vi "CapacitanceNavigation v2.1.vi"() -> ()   [LabVIEW 2021]
uses:
  <userlib>/Nanonis Prog Interface V5/Nanonis Prog Interface.lvlib
panel:
  in  "Z Frequency (Hz)":sgl=261.0
  in  "Z- Delta cap threshold (pA)":dbl=0.1
  in  "Z Amplitude (V)":sgl=260.0
  out "Delta reached?":bool
  out "Cap reached?":bool
  in  "Cap threshold (pA)":dbl
  in  "Z+ Delta cap threshold (pA)":dbl
  in  "pause":bool
  in  "Delete First Entry":bool
  in  "Time between averages (ms)":u32
  out "Avg index":i32=49
  in  "Averages":i32=50
  in  "milliseconds to wait":u32=1000
  in  "stop":bool
  in  "?":bool
  in  "Max Steps":u16=500
  in  "Direction":enum16{"X +", "X -", "Y +", "Y -", "Z +", "Z -"}(ring)=enum."Z +"
  out "Delta":cluster{"index":i32, sgl}[](graph)=[{"index"=100, -1.3574829}, {"index"=200, -1.4841919}, {"index"=300, -1.576477}, {"index"=400, -1.5935059}, {"index"=500, -1.618042}, {"index"=600, -1.6258545}, {"index"=700, -1.5469971}, {"index"=800, -1.4503174}, {"index"=900, -1.5161133}, {"index"=1000, -1.3947754}, {"index"=1100, -1.4649048}, {"index"=1200, -1.3322754}, {"index"=1300, -1.392456}, {"index"=1400, -1.2904053}, {"index"=1500, -1.291626}, {"index"=1600, -1.2921143}, {"index"=1700, -1.2836304}, {"index"=1800, -1.3444824}, {"index"=1900, -1.2155762}, {"index"=2000, -1.2328491}, {"index"=2100, -1.2090454}, {"index"=2200, -1.2058716}, {"index"=2300, -1.2508545}, {"index"=2400, -1.2296753}, {"index"=2500, -1.1306152}, {"index"=2600, -1.2440186}, {"index"=2700, -1.1461792}, {"index"=2800, -1.2349854}, {"index"=2900, -1.125}, {"index"=3000, -1.1894531}, {"index"=3100, -1.1911011}, {"index"=3200, -1.1334229}, {"index"=3300, -1.2139282}, {"index"=3400, -1.0455322}, {"index"=3500, -1.1482544}, {"index"=3600, -1.1663208}, {"index"=3700, -1.1547852}, {"index"=3800, -1.1334229}, {"index"=3900, -1.1394043}, {"index"=4000, -1.1153564}, {"index"=4100, -1.1187744}, {"index"=4200, -1.1342163}, {"index"=4300, -1.1434326}, {"index"=4400, -1.0510864}, {"index"=4500, -1.0391235}, {"index"=4600, -1.0696411}, {"index"=4700, -1.050354}, {"index"=4800, -1.09552}, {"index"=4900, -1.0064087}, {"index"=5000, -1.0879517}, {"index"=5100, -1.0756836}, {"index"=5200, -1.064331}, {"index"=5300, -1.0778809}, {"index"=5400, -1.0646973}, {"index"=5500, -1.0031738}, {"index"=5600, -1.0564575}, {"index"=5700, -1.0297852}, {"index"=5800, -0.9793091}, {"index"=5900, -1.0583496}, {"index"=6000, -1.0194702}, {"index"=6100, -0.9897461}, {"index"=6200, -0.99768066}, {"index"=6300, -1.0195312}, {"index"=6400, -0.9753418}, {"index"=6500, -1.0460205}, {"index"=6600, -0.9507446}, {"index"=6700, -0.9986572}, {"index"=6800, -0.9227295}, {"index"=6900, -0.90026855}, {"index"=7000, -0.96069336}, {"index"=7100, -0.92089844}, {"index"=7200, -0.9293823}, {"index"=7300, -0.85827637}, {"index"=7400, -0.94433594}, {"index"=7500, -0.8942871}, {"index"=7600, -0.91204834}, {"index"=7700, -0.9284668}, {"index"=7800, -0.994812}, {"index"=7900, -0.89501953}, {"index"=8000, -0.880188}, {"index"=8100, -0.95428467}, {"index"=8200, -0.8895874}, {"index"=8300, -0.951355}, {"index"=8400, -0.94384766}, {"index"=8500, -0.9460449}, {"index"=8600, -0.9188843}, {"index"=8700, -0.94177246}, {"index"=8800, -0.9863281}, {"index"=8900, -0.85375977}, {"index"=9000, -0.9229126}, {"index"=9100, -0.90771484}, {"index"=9200, -0.9472046}, {"index"=9300, -0.8875122}, {"index"=9400, -0.84661865}, {"index"=9500, -0.91223145}, {"index"=9600, -0.8786621}, {"index"=9700, -0.80389404}, {"index"=9800, -0.36602783}, {"index"=9900, 0.0076904297}, {"index"=10000, 0.010681152}, {"index"=10100, 0.0065307617}, {"index"=10200, -0.048583984}, {"index"=10300, 0.057373047}, {"index"=10400, 6.1035156e-05}, {"index"=10500, -0.085876465}]
  in  "Number of Steps":u16=100
  out "Capacitance":cluster{"index":i32, sgl}[](graph)=[{"index"=0, 783.6142}, {"index"=100, 782.2567}, {"index"=200, 780.7725}, {"index"=300, 779.19604}, {"index"=400, 777.60254}, {"index"=500, 775.9845}, {"index"=600, 774.35864}, {"index"=700, 772.81165}, {"index"=800, 771.3613}, {"index"=900, 769.8452}, {"index"=1000, 768.45044}, {"index"=1100, 766.98553}, {"index"=1200, 765.65326}, {"index"=1300, 764.2608}, {"index"=1400, 762.9704}, {"index"=1500, 761.6788}, {"index"=1600, 760.38666}, {"index"=1700, 759.103}, {"index"=1800, 757.75854}, {"index"=1900, 756.54297}, {"index"=2000, 755.3101}, {"index"=2100, 754.1011}, {"index"=2200, 752.8952}, {"index"=2300, 751.64435}, {"index"=2400, 750.4147}, {"index"=2500, 749.28406}, {"index"=2600, 748.04004}, {"index"=2700, 746.89386}, {"index"=2800, 745.6589}, {"index"=2900, 744.5339}, {"index"=3000, 743.3444}, {"index"=3100, 742.1533}, {"index"=3200, 741.0199}, {"index"=3300, 739.80597}, {"index"=3400, 738.76044}, {"index"=3500, 737.6122}, {"index"=3600, 736.44586}, {"index"=3700, 735.2911}, {"index"=3800, 734.15765}, {"index"=3900, 733.01825}, {"index"=4000, 731.9029}, {"index"=4100, 730.7841}, {"index"=4200, 729.6499}, {"index"=4300, 728.5065}, {"index"=4400, 727.4554}, {"index"=4500, 726.41626}, {"index"=4600, 725.3466}, {"index"=4700, 724.29626}, {"index"=4800, 723.20074}, {"index"=4900, 722.19434}, {"index"=5000, 721.1064}, {"index"=5100, 720.0307}, {"index"=5200, 718.9664}, {"index"=5300, 717.8885}, {"index"=5400, 716.8238}, {"index"=5500, 715.8206}, {"index"=5600, 714.76416}, {"index"=5700, 713.7344}, {"index"=5800, 712.75507}, {"index"=5900, 711.6967}, {"index"=6000, 710.67725}, {"index"=6100, 709.6875}, {"index"=6200, 708.6898}, {"index"=6300, 707.6703}, {"index"=6400, 706.69495}, {"index"=6500, 705.6489}, {"index"=6600, 704.6982}, {"index"=6700, 703.6995}, {"index"=6800, 702.7768}, {"index"=6900, 701.8765}, {"index"=7000, 700.91583}, {"index"=7100, 699.99493}, {"index"=7200, 699.06555}, {"index"=7300, 698.2073}, {"index"=7400, 697.26294}, {"index"=7500, 696.36865}, {"index"=7600, 695.4566}, {"index"=7700, 694.52814}, {"index"=7800, 693.5333}, {"index"=7900, 692.6383}, {"index"=8000, 691.7581}, {"index"=8100, 690.80383}, {"index"=8200, 689.91425}, {"index"=8300, 688.9629}, {"index"=8400, 688.01904}, {"index"=8500, 687.073}, {"index"=8600, 686.1541}, {"index"=8700, 685.21234}, {"index"=8800, 684.226}, {"index"=8900, 683.37225}, {"index"=9000, 682.44934}, {"index"=9100, 681.5416}, {"index"=9200, 680.5944}, {"index"=9300, 679.7069}, {"index"=9400, 678.8603}, {"index"=9500, 677.94806}, {"index"=9600, 677.0694}, {"index"=9700, 676.2655}, {"index"=9800, 675.8995}, {"index"=9900, 675.90717}, {"index"=10000, 675.91785}, {"index"=10100, 675.9244}, {"index"=10200, 675.8758}, {"index"=10300, 675.93317}, {"index"=10400, 675.9332}, {"index"=10500, 675.84735}]
  in  "XY Frequency (Hz)":sgl=261.0
  in  "XY Amplitude (V)":sgl=300.0
  # "KPN: CORRECT NAVIGATION PROGRAM, 6/12/22"
  # "Threshold only works \nin Z+ direction"
  # "Max Steps On"
  # "Max Steps Off"
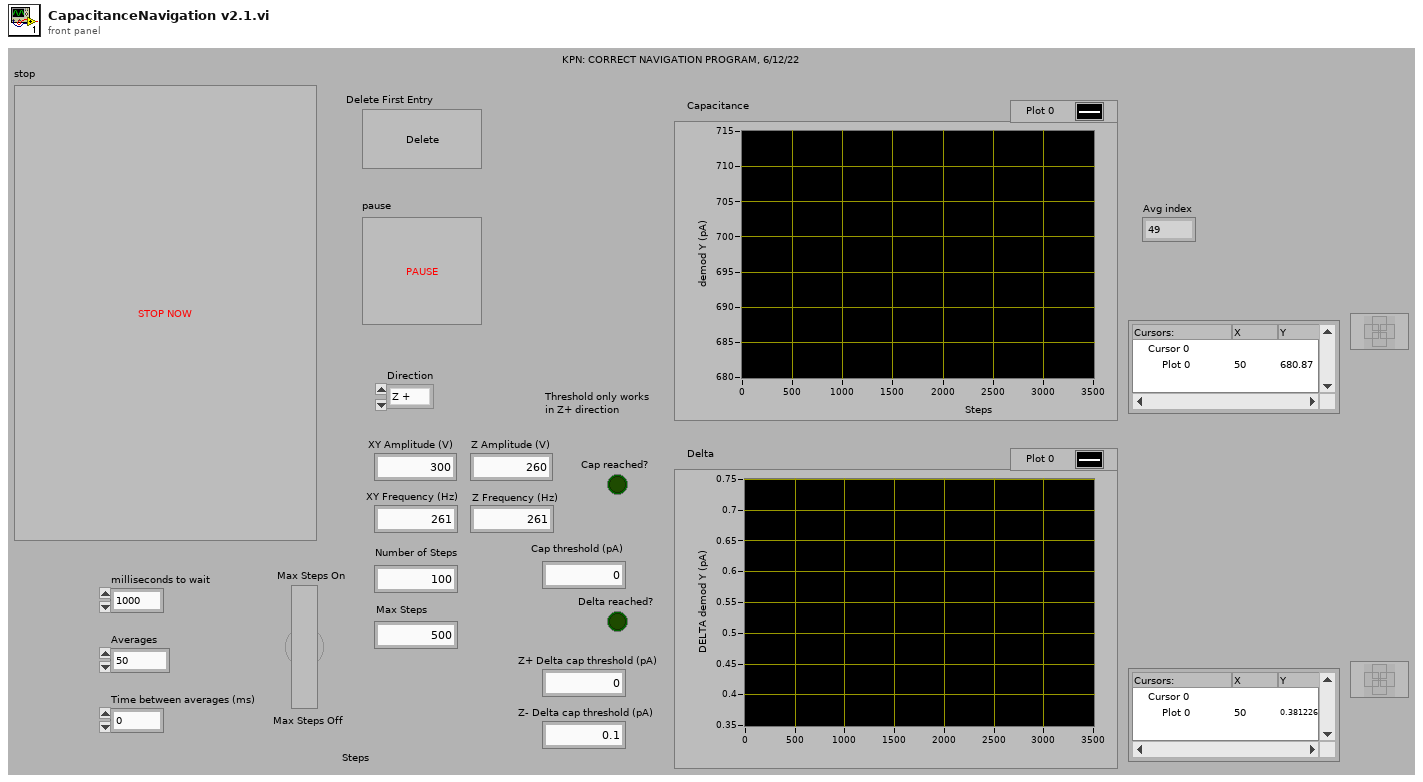
[diagram p1: front panel]
types:
  T1 = enum8{"Group 1", "Group 2", "Group 3", "Group 4", "Group 5", "Group 6"}
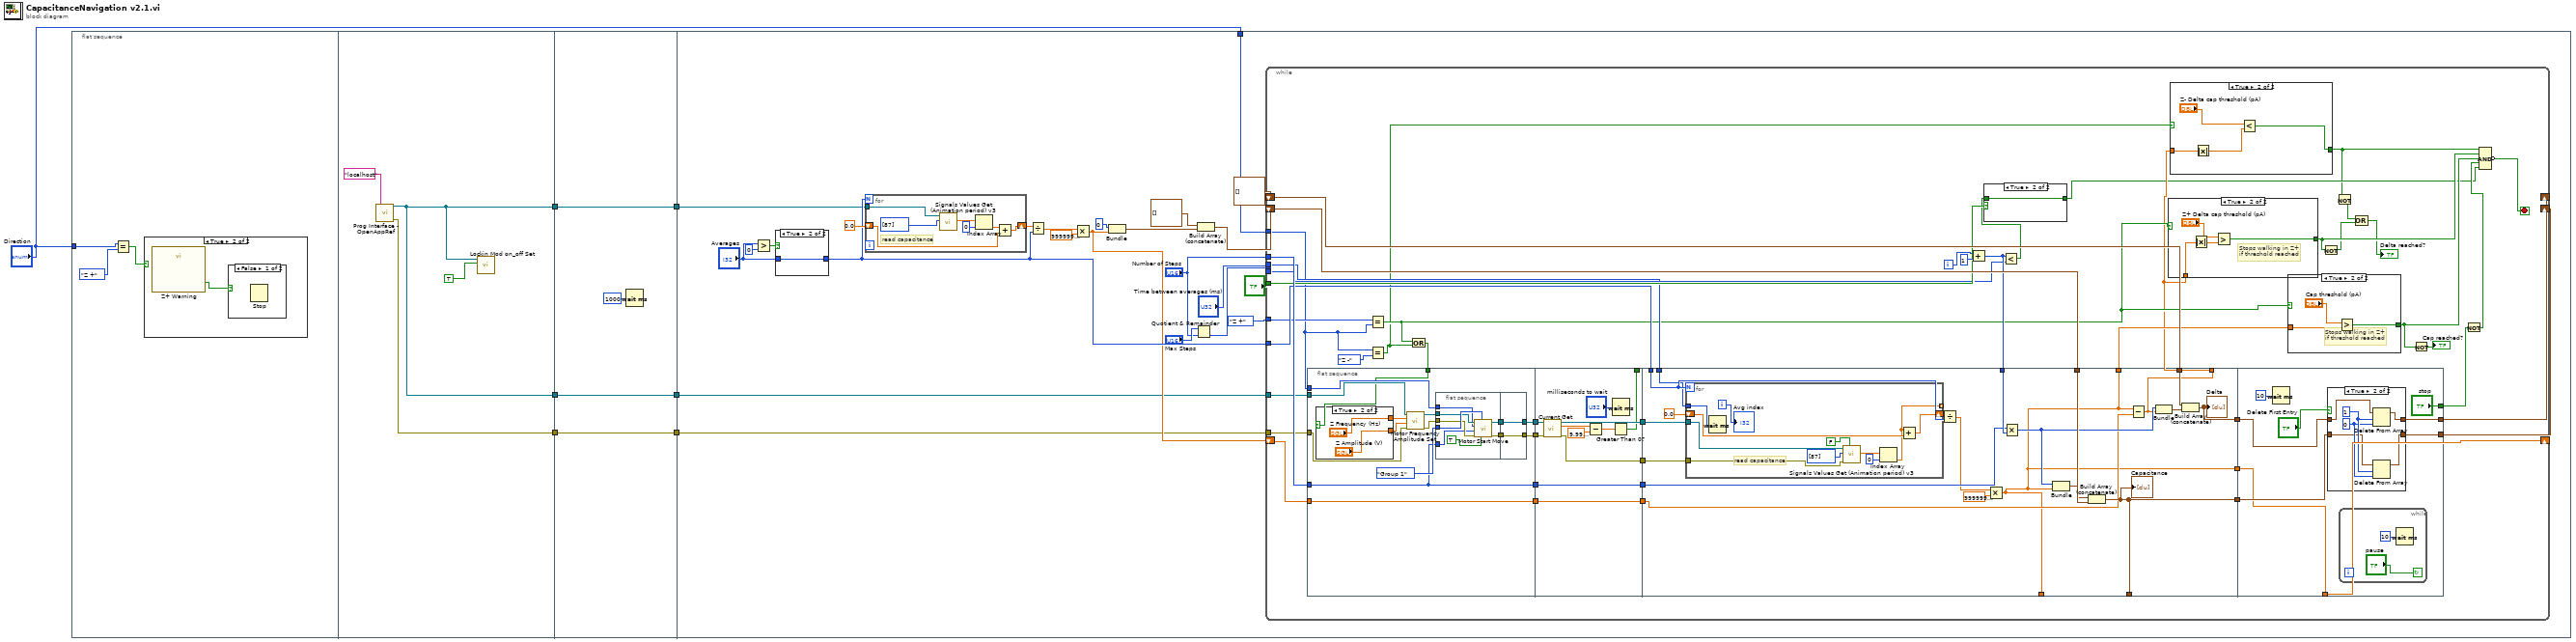
[diagram p0: block diagram]
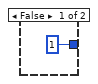
[diagram p4: hidden frame]
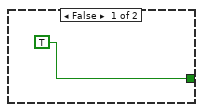
[diagram p5: hidden frame]
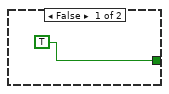
[diagram p6: hidden frame]
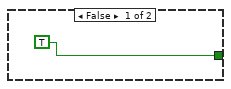
[diagram p7: hidden frame]
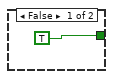
[diagram p8: hidden frame]
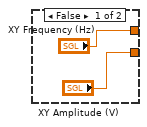
[diagram p9: hidden frame]
diagram:
  n1 = flat-sequence {
    tunnel: "Direction" -> [w10]
    tunnel: [w15] -> w7
    tunnel: [w13] -> w5
    tunnel: [w13] -> w3
    tunnel: w7 -> [w19]
    tunnel: [w19] -> w6
    tunnel: w5 -> [w18]
    tunnel: [w18] -> w4
    tunnel: w3 -> [w17]
    tunnel: [w17] -> w2
    tunnel: w6 -> [w23]
    tunnel: w4 -> [w22]
    tunnel: w2 -> [w21]
    tunnel: "Direction" -> [w20]
    frame #0 {
      n2 = Equal?(x=w10, y=enum16{"X +", "X -", "Y +", "Y -", "Z +", "Z -"}."Z +") -> (x = y?=w8:bool)
      n3 = case shown="True" w8 {
        frame False {
        }
        frame True {
          n4 = call "Z+ Warning"() -> ("OK"=w11:bool)  [unwired: 18 in, 1 out]
          n5 = case shown="False" w11 {
            frame False {
              n6 = Stop() -> ()  [unwired: 1 in]
            }
            frame True {
            }
          }
        }
      }
    }
    frame #1 {
      n7 = call <userlib>:"Prog Interface - OpenAppRef.vi"("Machine name (local machine IP)"="localhost" ("machine name (localhost)")) -> ("Error out"=w15:errorcluster, "Application reference"=w13:refnum<vi>)  [unwired: 5 in]
      n8 = call <userlib>:"Lockin Mod on_off Set.vi"("Lockin ON/OFF"=TRUE, "Application ref in"=w13) -> ()  [unwired: 8 in, 2 out]
    }
    frame #2 {
      n9 = Wait (ms)(milliseconds to wait=u32 1000) -> ()  [unwired: 1 out]
    }
    frame #3 {
      n10 = Greater?(x="Averages", y=0) -> (0:w32:bool)
      n11 = case shown="True" w32 {
        tunnel: "Averages" -> [_ w52]
        tunnel: [1 ("Averages") w52] -> w27
        frame False {
        }
        frame True {
        }
      }
      n12 = for {
        N: w27 -> [_]
        shift-right: [w45] -> w28
        shift-left: sgl 0.0 ("Internal Ch Value") -> [w47]
        tunnel: w22 -> [w44]
        # "read capacitance"
        n13 = call <userlib>:"Signals Values Get (Animation period) v3.vi"("Signals indexes (0-127)"=i8[] [87], "Application ref in"=w44) -> ("Signals Values"=w48:sgl[])  [unwired: 6 in, 2 out]
        n14 = Index Array(array=w48, index=0) -> (element=w46:sgl)
        n15 = Add(x=w46, y=w47) -> (x+y=w45:sgl)
      }
      n16 = Divide(x=w28, y=w27) -> (x/y=w26:sgl)
      n17 = Multiply(x=w26, y=sgl 1000000000000.0) -> (x*y=w25:sgl)
      n18 = Bundle("index"=0, w25) -> (w41:cluster{"index":i32, sgl})  [unwired: 1 in]
      n19 = Quotient & Remainder(x="Max Steps", y="Number of Steps") -> (floor(x/y)=w35:u16)  [unwired: 1 out]
      n20 = Build Array (concatenate)(cluster{i32, sgl}[] [], w41) -> (w40:cluster{"index":i32, sgl}[])
      n21 = while {
        shift-right: [w78] -> _
        shift-left: w40 -> [w97]
        shift-right: [w90] -> _
        shift-left: cluster{i32, sgl}[] [] -> [w89]
        tunnel: w20 -> [w69]
        tunnel: "Number of Steps" -> [w88]
        tunnel: w35 -> [w83]
        tunnel: "?" -> [w87]
        tunnel: w27 -> [w81]
        tunnel: "Time between averages (ms)" -> [w80]
        shift-right: [w76] -> _
        shift-left: w25 -> [w75]
        tunnel: enum16{"X +", "X -", "Y +", "Y -", "Z +", "Z -"}."Z +" ("Direction") -> [w70]
        tunnel: w23 -> [w54]
        tunnel: w21 -> [w53]
        i -> [w86]
        stop <- w60 stop-if-true
        n22 = flat-sequence {
          tunnel: [w120] -> w99
          tunnel: w53 -> [w123]
          tunnel: w54 -> [w126]
          tunnel: [w125] -> w95
          tunnel: [w124] -> w94
          tunnel: w69 -> [w119]
          tunnel: w88 -> [w120]
          tunnel: w75 -> [w118]
          tunnel: [w118] -> w74
          tunnel: w66 -> [w117]
          tunnel: w99 -> [w155]
          tunnel: [w155] -> w98
          tunnel: w95 -> [w154]
          tunnel: w94 -> [w153]
          tunnel: [w152] -> w93
          tunnel: [w151] -> w92
          tunnel: [w148] -> _
          tunnel: w74 -> [w145]
          tunnel: [w145] -> w73
          tunnel: [w159] -> _
          tunnel: w84 -> [w174]
          tunnel: w98 -> [w171]
          tunnel: w97 -> [w172]
          tunnel: [w156] -> _
          tunnel: w93 -> [w170]
          tunnel: w92 -> [w169]
          tunnel: [w165] -> w91
          tunnel: w89 -> [w166]
          tunnel: w81 -> [w161]
          tunnel: w80 -> [w160]
          tunnel: [w159] -> w79
          tunnel: [w156] -> w77
          tunnel: w73 -> [w158]
          tunnel: [w157] -> w61
          tunnel: [w156] -> w72
          tunnel: w91 -> [w192]
          tunnel: [w191] -> w90
          tunnel: ["stop"] -> w82
          tunnel: [w189] -> w78
          tunnel: w79 -> [w190]
          tunnel: w77 -> [w188]
          tunnel: [w188] -> w76
          frame #0 {
            n23 = case shown="True" w117 {
              tunnel: ["XY Amplitude (V)" "Z Amplitude (V)"] -> w129
              tunnel: ["XY Frequency (Hz)" "Z Frequency (Hz)"] -> w116
              frame False {
              }
              frame True {
              }
            }
            n24 = call <userlib>:"Motor Frequency Amplitude Set.vi"("Error in (no error)"=w126, "Amplitude (V) (NaN=no change)"=w129, "Frequency (Hz) (NaN=no change)"=w116, "Application ref in"=w123) -> ("Error out"=w127:errorcluster, "Application ref out"=w128:refnum<vi>)  [unwired: 6 in]
            n25 = flat-sequence {
              tunnel: T1."Group 1" ("Group") -> [w141]
              tunnel: w128 -> [w140]
              tunnel: w127 -> [w139]
              tunnel: w120 -> [w138]
              tunnel: [w137] -> w122
              tunnel: [w136] -> w121
              tunnel: w119 -> [w135]
              tunnel: [w143] -> w124
              tunnel: [w144] -> w125
              tunnel: w122 -> [w144]
              tunnel: w121 -> [w143]
              frame #0 {
                n26 = call <userlib>:"Motor Start Move.vi"("Wait until finished? (F)"=TRUE, "Group"=w141, "Error in (no error)"=w139, "Number of steps"=w138, "Direction"=w135, "Application ref in"=w140) -> ("Error out"=w136:errorcluster, "Application ref out"=w137:refnum<vi>)  [unwired: 3 in]
              }
              frame #1 {
              }
            }
          }
          frame #1 {
            n27 = call <userlib>:"Current Get.vi"("Error in (no error)"=w153, "Application ref in"=w154) -> ("Error out"=w152:errorcluster, "Current (A)"=w150:sgl, "Application ref out"=w151:refnum<vi>)  [unwired: 5 in]
            n28 = Subtract(x=w150, y=sgl 1e-09) -> (x-y=w149:sgl)
            n29 = Greater Than 0?(x=w149) -> (x > 0?=w148:bool)
            n30 = Wait (ms)(milliseconds to wait="milliseconds to wait") -> ()  [unwired: 1 out]
          }
          frame #2 {
            n31 = for {
              N: w161 -> [_]
              tunnel: w170 -> [w183]
              tunnel: w169 -> [w182]
              shift-right: [w180] -> w163
              shift-left: sgl 0.0 ("y") -> [w181]
              tunnel: w160 -> [w178]
              tunnel: [w176] -> _ mode=indexing
              i -> [w179]
              # "read capacitance"
              n32 = Wait (ms)(milliseconds to wait=w178) -> ()  [unwired: 1 out]
              n33 = call <userlib>:"Signals Values Get (Animation period) v3.vi"("Wait for newest data (F=False)"=FALSE, "error in (no error)"=w183, "Signals indexes (0-127)"=i8[] [87], "Application ref in"=w182) -> ("Signals Values"=w184:sgl[])  [unwired: 4 in, 2 out]
              n34 = Index Array(array=w184, index=0) -> (element=w176:sgl)
              n35 = Add(x=w176, y=w181) -> (x+y=w180:sgl)
              "Avg index" <- w179
            }
            n36 = Divide(x=w163, y=w161) -> (x/y=w162:sgl)
            n37 = Multiply(x=w162, y=sgl 1000000000000.0) -> (x*y=w156:sgl)
            n38 = Multiply(x=w171, y=w174) -> (x*y=w168:i32)
            n39 = Bundle(w168, w156) -> (w173:cluster{i32, sgl})  [unwired: 1 in]
            n40 = Build Array (concatenate)(w172, w173) -> (w159:cluster{"index":i32, sgl}[])
            "Capacitance" <- w159
            n41 = Subtract(x=w156, y=w158) -> (x-y=w157:sgl)
            n42 = Bundle(w168, w157) -> (w167:cluster{i32, sgl})  [unwired: 1 in]
            n43 = Build Array (concatenate)(w166, w167) -> (w165:cluster{i32, sgl}[])
            "Delta" <- w165
          }
          frame #3 {
            n44 = Wait (ms)(milliseconds to wait=u32 10) -> ()  [unwired: 1 out]
            n45 = case shown="True" "Delete First Entry" {
              tunnel: w192 -> [w198 w202]
              tunnel: [w198 w201] -> w191
              tunnel: w190 -> [w197 w199]
              tunnel: [w197 w200] -> w189
              frame False {
              }
              frame True {
                w204 = 1 ("length")
                w203 = 0 ("index")
                n46 = Delete From Array(array=w202, length=w204, index=w203) -> (array with subset deleted=w201:cluster{i32, sgl}[])  [unwired: 1 out]
                n47 = Delete From Array(array=w199, length=w204, index=w203) -> (array with subset deleted=w200:cluster{"index":i32, sgl}[])  [unwired: 1 out]
              }
            }
            n48 = while {
              stop <- "pause" continue-if-true
              n49 = Wait (ms)(milliseconds to wait=u32 10) -> ()  [unwired: 1 out]
            }
          }
        }
        n50 = Equal?(x=w70, y=w69) -> (x = y?=w67:bool)
        n51 = Equal?(x=w69, y=enum16{"X +", "X -", "Y +", "Y -", "Z +", "Z -"}."Z -") -> (x = y?=w65:bool)
        n52 = Or(x=w67, y=w65) -> (x .or. y?=w66:bool)
        n53 = Add(x=w86, y=u16 1) -> (x+y=w84:i32)
        n54 = Less?(x=w84, y=w83) -> (x < y?=w85:bool)
        n55 = case shown="True" w87 {
          tunnel: w85 -> [_ w115]
          tunnel: [TRUE w115] -> w59
          frame False {
          }
          frame True {
          }
        }
        n56 = case shown="True" w67 {
          tunnel: w61 -> [_ w113]
          tunnel: [TRUE w111] -> w64
          frame False {
          }
          frame True {
            # "Stops walking in Z+ \nif threshold reached"
            n57 = Absolute Value(x=w113) -> (abs(x)=w110:sgl)
            n58 = Greater?(x="Z+ Delta cap threshold (pA)", y=w110) -> (0:w111:bool)
          }
        }
        n59 = case shown="True" w65 {
          tunnel: [TRUE w102] -> w57
          tunnel: w61 -> [_ w104]
          frame False {
          }
          frame True {
            n60 = Absolute Value(x=w104) -> (abs(x)=w103:sgl)
            n61 = Less?(x="Z- Delta cap threshold (pA)", y=w103) -> (x < y?=w102:bool)
          }
        }
        n62 = case shown="True" w67 {
          tunnel: w72 -> [_ w107]
          tunnel: [TRUE w106] -> w63
          frame False {
          }
          frame True {
            # "Stops walking in Z+ \nif threshold reached"
            n63 = Greater?(x="Cap threshold (pA)", y=w107) -> (0:w106:bool)
          }
        }
        n64 = Not(x=w64) -> (.not. x?=w58:bool)
        n65 = Not(x=w57) -> (.not. x?=w55:bool)
        n66 = Compound Arithmetic op=OR(w55, w58) -> (→"Delta reached?":bool)
        n67 = Not(x=w63) -> (.not. x?=→"Cap reached?":bool)
        n68 = Not(x=w82) -> (.not. x?=w62:bool)
        n69 = Compound Arithmetic op=AND(w57, w64, w63, w62, w59) -> (invert w60:bool)
      }
    }
  }
